vi "View Camera.vi"() -> ()   [LabVIEW 2013]
uses:
  ROS/Code/SubVIs/BaxterCamera.ctl
panel:
  in  "[user-specified font]":T1={"Font Name:"="Arial Black", "Size"=60, "Strikeout?"=FALSE, "Italic?"=FALSE, "Underline?"=FALSE, "Outline?"=FALSE, "Shadow?"=FALSE, "Bold?"=TRUE}
  in  "origin":cluster{"x":i16, "y":i16}={"x"=50, "y"=420}
  in  "String":string
  in  "Display":bool
  in  "Save":bool
  in  "stop":bool
  in  "Camera":T2=enum."right_hand_camera"
  out "picture":picture
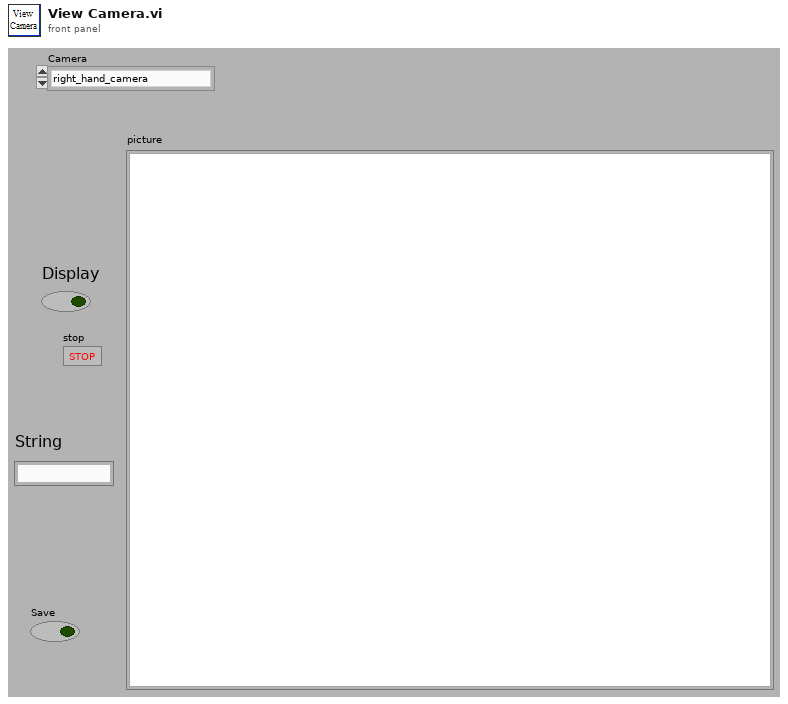
[diagram p1: front panel]
types:
  T1 = cluster{"Font Name:":string, "Size":i16, "Strikeout?":bool, "Italic?":bool, "Underline?":bool, "Outline?":bool, "Shadow?":bool, "Bold?":bool}
  T2 = typedef "BaxterCamera.ctl" = enum16{"left_hand_camera", "right_hand_camera", "head_camera"}
  T3 = enum16{"User-specified Font", "Application Font", "System Font", "Dialog Font"}
  T4 = cluster{"left":i16, "top":i16, "right":i16, "bottom":i16}
  T5 = typedef "imagedata.ctl" = cluster{"image type":i32, "image depth":i32, "image":u8[], "mask":u8[], "colors":u32[], "Rectangle":cluster{"left":i16, "top":i16, "right":i16, "bottom":i16}}
  T6 = typedef "LVBoundsTypeDef.ctl" = cluster{"Width":u32, "Height":u32}
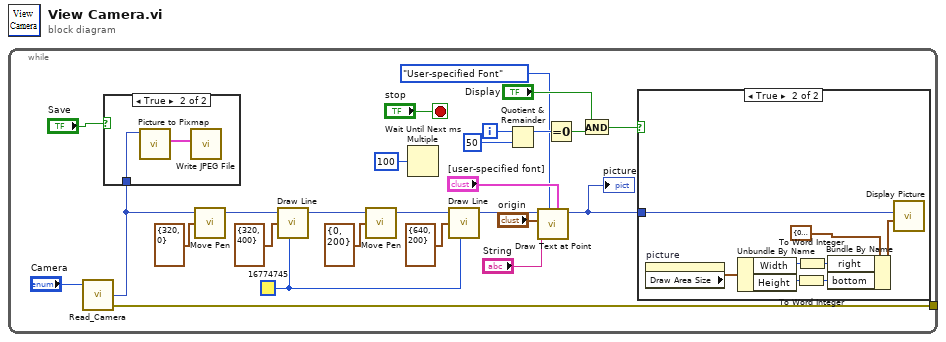
[diagram p0: block diagram]
diagram:
  n1 = while {
    tunnel: [w24] -> _
    i -> [w12]
    stop <- "stop" stop-if-true
    w6 = u32 16774745
    n2 = call "Read_Camera.vi"("Camera"="Camera") -> ("picture"=w14:picture, "error out"=w24:errorcluster)  [unwired: 2 in, 3 out]
    n3 = case shown="True" "Save" {
      tunnel: w14 -> [_ w36]
      frame False {
      }
      frame True {
        n4 = call <vilib>:"Picture to Pixmap.vi"("picture"=w36) -> ("image data"=w35:T5)  [unwired: 9 in, 1 out]
        n5 = call <vilib>:"Write JPEG File.vi"("image data"=w35) -> ()  [unwired: 9 in, 2 out]
      }
    }
    n6 = call <vilib>:"Move Pen.vi"("new position"=cluster{"x":i16, "y":i16} {"x"=320, "y"=0}, "picture"=w14) -> ("new picture"=w21:picture)  [unwired: 3 in]
    n7 = call <vilib>:"Draw Line.vi"("picture"=w21, "end point"=cluster{"x":i16, "y":i16} {"x"=320, "y"=400}, "color(black)"=w6) -> ("new picture"=w15:picture)  [unwired: 6 in]
    n8 = call <vilib>:"Move Pen.vi"("new position"=cluster{"x":i16, "y":i16} {"x"=0, "y"=200}, "picture"=w15) -> ("new picture"=w18:picture)  [unwired: 3 in]
    n9 = Wait Until Next ms Multiple(millisecond multiple=u32 100) -> ()  [unwired: 1 out]
    n10 = call <vilib>:"Draw Line.vi"("picture"=w18, "end point"=cluster{"x":i16, "y":i16} {"x"=640, "y"=200}, "color(black)"=w6) -> ("new picture"=w13:picture)  [unwired: 6 in]
    n11 = Quotient & Remainder(x=w12, y=50) -> (x-y*floor(x/y)=w10:i32)  [unwired: 1 out]
    n12 = call <vilib>:"Draw Text at Point.vi"("[user-specified font]"="[user-specified font]", "desired font(Application)"=T3."User-specified Font", "text"="String", "origin"="origin", "picture"=w13) -> ("new picture"=w1:picture)  [unwired: 5 in, 1 out]
    "picture" <- w1
    n13 = Equal To 0?(x=w10) -> (x = 0?=w9:bool)
    n14 = And(x="Display", y=w9) -> (x .and. y?=w7:bool)
    n15 = case shown="True" w7 {
      tunnel: w1 -> [_ w28]
      frame False {
      }
      frame True {
        n16 = property on="picture" class="Pict"() -> ("Draw Area Size"=w34:T6)  [unwired: 2 in, 2 out]
        n17 = Unbundle By Name(w34) -> ("Width"=w32:u32, "Height"=w31:u32)
        n18 = To Word Integer(number=w31) -> (16bit integer=w29:i16)
        n19 = To Word Integer(number=w32) -> (16bit integer=w30:i16)
        n20 = Bundle By Name(cluster=T4 {"left"=0, "top"=0, "right"=640, "bottom"=400} ("rect"), "right"=w30, "bottom"=w29) -> (w27:T4)
        n21 = call "Display Picture.vi"("rect"=w27, "picture"=w28) -> ()  [unwired: 9 in, 1 out]
      }
    }
  }
